vi "Find Related Entities.vi"(7 "Entity Type":refnum<class "Entity.lvclass">, 8 "error in (no error)":errorcluster, 9 "Relation":T1, 10 "Primary ID":T3, 11 "Entity Manager in":refnum<class "Entity Manager.lvclass">) -> (0 "error out":errorcluster, 2 "Entities":refnum<class "Entity.lvclass">[](array[class]), 3 "Entity Manager out":refnum<class "Entity Manager.lvclass">)   [LabVIEW 2020, in "Conditu2.lvlib" / "Entity Manager.lvclass"]
uses:
  Entity Manager.lvclass
  Entity/Entity.lvclass
  Entity ID.ctl
  Columns/Relation/Relation Info.ctl
  Relation Mapping.ctl
  Entity Manager.lvclass/Entity Manager.ctl
  Database Platform/Database Platform.lvclass
  Conditu2.lvlib
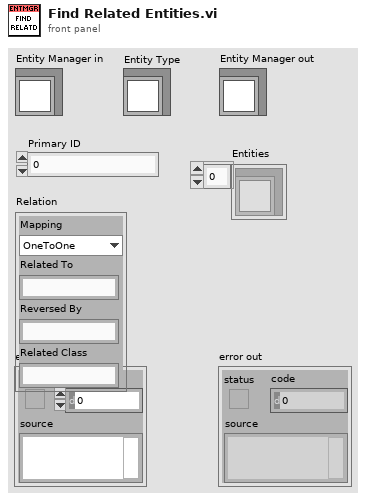
[diagram p1: front panel]
types:
  T1 = typedef "Conditu2.lvlib/Relation Info.ctl" = cluster{"Mapping":T2, "Related To":string, "Reversed By":string, "Related Class":string}
  T2 = typedef "Conditu2.lvlib/Relation Mapping.ctl" = enum16{"OneToOne", "OneToMany", "ManyToOne", "ManyToMany"}
  T3 = typedef "Conditu2.lvlib/Entity ID.ctl" = i64
  T4 = typedef "Conditu2.lvlib/Entity Manager.lvclass/Entity Info.ctl" = cluster{"Entity":refnum<class "Entity.lvclass">, "Types":refnum<class "Type.lvclass">[], "Type Name Map":map{string, i32}, "Has Relation":bool}
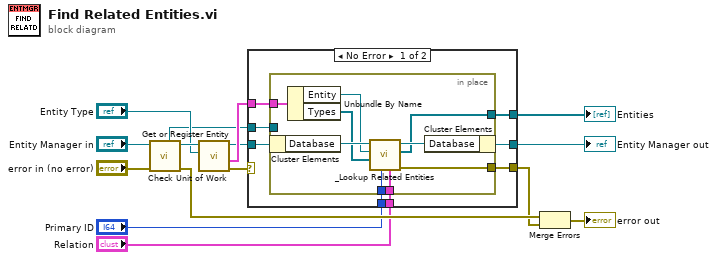
[diagram p0: block diagram]
diagram:
  n1 = call "Check Unit of Work.vi"("error in (no error)"="error in (no error)", "Entity Manager in"="Entity Manager in") -> ("error out"=w15:errorcluster, "Entity Manager out"=w12:refnum<class "Entity Manager.lvclass">, "Unit Of Work"=w7:refnum<class "Unit Of Work Session.lvclass">)  [unwired: 7 in]
  n2 = call "Get or Register Entity.vi"("Entity"="Entity Type", "Entity Manager in"=w12) -> ("error out"=w10:errorcluster, "Entity Info"=w9:T4, "Entity Manager out"=w8:refnum<class "Entity Manager.lvclass">)  [unwired: 7 in]
  n3 = case shown="No Error" w10 {
    selector: w10 -> [_ w33]
    tunnel: w9 -> [w21 _]
    tunnel: w8 -> [w23 w34]
    tunnel: w7 -> [w22 _]
    tunnel: [w20 w34] -> w6
    tunnel: [w16 w33] -> w4
    tunnel: "Primary ID" -> [w19 _]
    tunnel: "Relation" -> [w18 _]
    tunnel: [w17 _] -> w1
    frame No Error {
      n4 = in-place {
        in-place-border: w22 -> [_]
        in-place-border: w21 -> [w32]
        in-place-border: w19 -> [w29]
        in-place-border: w18 -> [w28]
        in-place-border: [w25] -> w17
        in-place-border: [w24] -> w16
        n5 = in-place-cluster #1(w23) -> ("Database"=w31:refnum<class "Database Platform.lvclass">)
        n6 = Unbundle By Name(w32) -> ("Entity"=w26:refnum<class "Entity.lvclass">, "Types"=w27:refnum<class "Type.lvclass">[])
        n7 = call "_Lookup Related Entities.vi"("Relation"=w28, "Primary ID"=w29, "Types"=w27, "Entity"=w26, "Database in"=w31) -> ("error out"=w24:errorcluster, "Entities"=w25:refnum<class "Entity.lvclass">[], "Database out"=w30:refnum<class "Database Platform.lvclass">)  [unwired: 4 in]
        n8 = in-place-cluster #1("Database"=w30) -> (w20:refnum<class "Entity Manager.lvclass">)
      }
    }
    frame Error {
    }
  }
  "Entity Manager out" <- w6
  "Entities" <- w1
  n9 = Merge Errors(w15, w4) -> (→"error out":errorcluster)
